vi "Convex Hull 3D (GiftWrap).vi"(0 "Vertices":sgl[][](array[numeric])=[[0.0, 0.0, 0.0], [1.0, 0.0, 0.0], [1.0, 1.0, 0.0], [0.0, 1.0, 0.0], [0.0, 0.0, 1.0], [1.0, 0.0, 1.0], [1.0, 1.0, 1.0], [0.0, 1.0, 1.0], [10.0, 10.0, 0.0], [11.0, 10.0, 0.0], [11.0, 11.0, 0.0], [10.0, 11.0, 0.0], [10.0, 10.0, 1.0], [11.0, 10.0, 1.0], [11.0, 11.0, 1.0], [10.0, 11.0, 1.0]]) -> (1 "Convex hull triangles (partial proc.)":T1[](array[typedef]), 2 "Stack error":errorcluster)   [LabVIEW 2014]
uses:
  Typedefs/Triangle.ctl
  Typedefs/Edge.ctl
  Subroutines/Cross product 3D.vi
  Subroutines/Unit vector.vi
panel:
  # "PN 21/03/2015"
  # "Vertices"
  # "Edges"
  # "Unit normal"
  # "Edge unit normals"
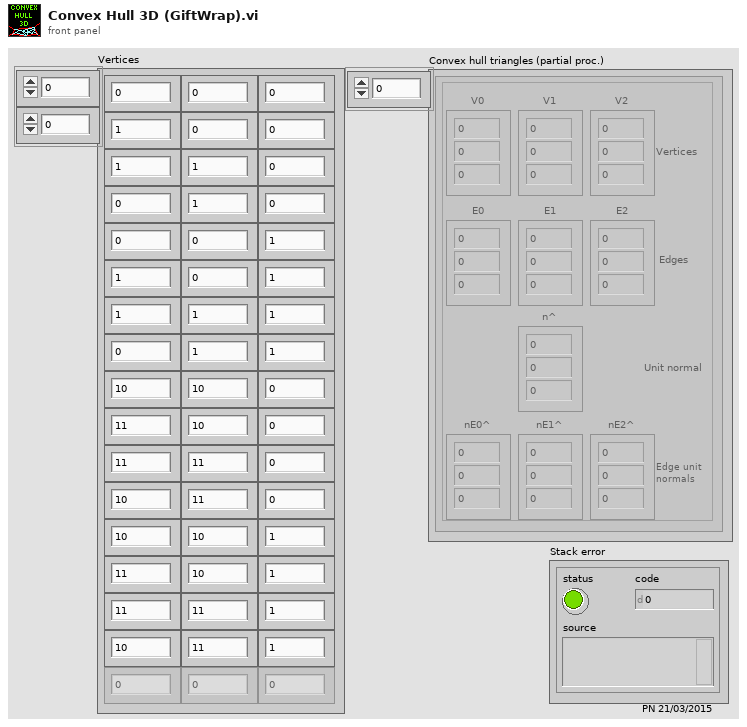
[diagram p1: front panel]
types:
  T1 = typedef "Triangle.ctl" = cluster{"V0":sgl[], "V1":sgl[], "V2":sgl[], "E0":sgl[], "E1":sgl[], "E2":sgl[], "n^":sgl[], "nE0^":sgl[], "nE1^":sgl[], "nE2^":sgl[]}
  T2 = typedef "Edge.ctl" = cluster{"V0":sgl[], "V1":sgl[], "E01":sgl[]}
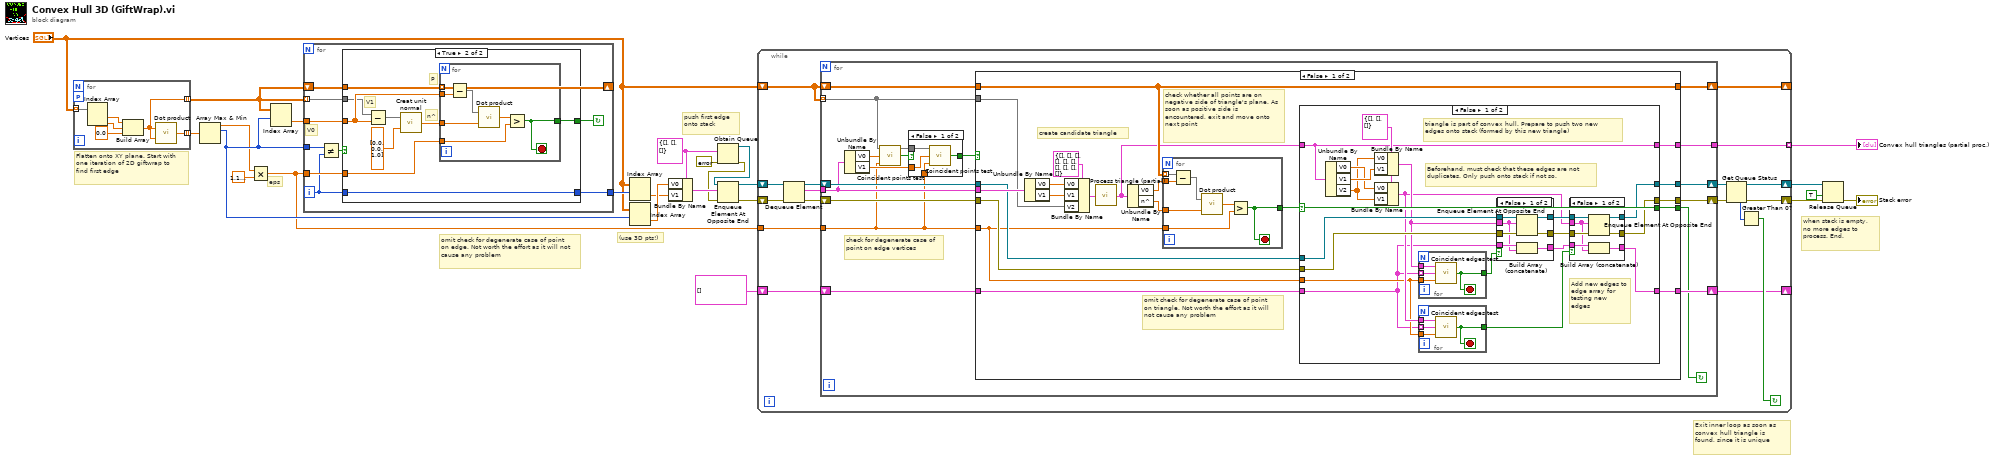
[diagram p0: block diagram]
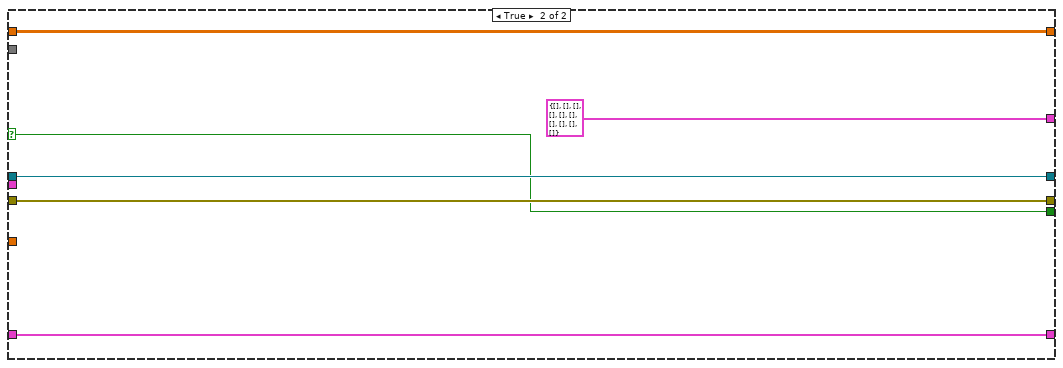
[diagram p6: hidden frame]
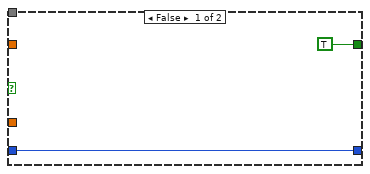
[diagram p7: hidden frame]
diagram:
  w12 = T2 {"V0"=[], "V1"=[], "E01"=[]} ("Edge")
  # "omit check for degenerate case of point on edge. Not worth the effort as it will not cause any problem"
  # "when stack is empty, no more edges to process. End."
  # "Exit inner loop as soon as convex hull triangle is found, since it is unique"
  # "(use 3D pts!)"
  # "push first edge onto stack"
  # "eps"
  # "Flatten onto XY plane. Start with one iteration of 2D giftwrap to find first edge"
  n1 = for {
    tunnel: "Vertices" -> [w30] mode=indexing
    tunnel: [w29] -> w24 mode=indexing
    workers-P: _ -> [_]
    tunnel: [w26] -> w22 mode=indexing
    n2 = Index Array(array=w30) -> (element #1=w28:sgl, element #2=w27:sgl)  [unwired: 2 in]
    n3 = Build Array(w28, w27, sgl 0.0 ("element")) -> (w26:sgl[])
    n4 = call "Dot product.vi"("B"=w26, "A"=w26) -> ("A . B"=w29:sgl)
  }
  n5 = Array Max & Min(array=w24) -> (max value=w4:sgl, max index (indices)=w13:i32)  [unwired: 2 out]
  n6 = Multiply(x=w4, y=sgl 1.1920929e-07) -> (x*y=w5:sgl)
  n7 = Index Array(array=w22, index (row)=w13) -> (element=w23:sgl[])  [unwired: 1 in]
  n8 = for {
    tunnel: w23 -> [w39]
    tunnel: w22 -> [w36] mode=indexing
    shift-right: [w37] -> _
    shift-left: w22 -> [w37]
    tunnel: w5 -> [w38]
    tunnel: [w33] -> w21
    tunnel: w13 -> [w31]
    i -> [w32]
    stop <- w35 continue-if-true
    # "V0"
    n9 = Not Equal?(x=w31, y=w32) -> (x != y?=w34:bool)
    n10 = case shown="True" w34 {
      tunnel: w39 -> [_ w48]
      tunnel: w38 -> [_ w47]
      tunnel: w37 -> [_ w46]
      tunnel: w36 -> [_ w45]
      tunnel: [TRUE w44] -> w35
      tunnel: w32 -> [w40 w42]
      tunnel: [w40 w42] -> w33
      frame False {
      }
      frame True {
        # "P"
        # "n^"
        # "V1"
        n11 = Subtract(x=w45, y=w48) -> (x-y=w43:sgl[])
        n12 = call "Creat unit normal.vi"("E2"=sgl[] [0.0, 0.0, 1.0], "E1"=w43) -> ("n^ = (E1 x E2) / ||E1 x E2||"=w49:sgl[])
        n13 = for {
          tunnel: w49 -> [w57]
          tunnel: w46 -> [w56] mode=indexing
          tunnel: w48 -> [w55]
          tunnel: w47 -> [w54]
          tunnel: [w53] -> w44
          stop <- w53 stop-if-true
          n14 = Subtract(x=w56, y=w55) -> (x-y=w52:sgl[])
          n15 = call "Dot product.vi"("B"=w57, "A"=w52) -> ("A . B"=w51:sgl)
          n16 = Greater?(x=w51, y=w54) -> (0:w53:bool)
        }
      }
    }
  }
  n17 = Index Array(array="Vertices", index (row)=w21) -> (element=w10:sgl[])  [unwired: 1 in]
  n18 = Index Array(array="Vertices", index (row)=w13) -> (element=w11:sgl[])  [unwired: 1 in]
  n19 = Bundle By Name(cluster=w12, "V0"=w11, "V1"=w10) -> (w18:T2)
  n20 = Obtain Queue(element data type=w12, error in (no error)=errorcluster {"status"=FALSE, "code"=0, "source"=""}) -> (queue out=w19:refnum<queue>, error out=w16:errorcluster)  [unwired: 3 in, 1 out]
  n21 = Enqueue Element At Opposite End(queue=w19, element=w18, error in (no error)=w16) -> (queue out=w8:refnum<queue>, error out=w9:errorcluster)  [unwired: 1 in, 1 out]
  n22 = while {
    shift-right: [w69] -> _
    shift-left: "Vertices" -> [w71]
    shift-right: [w65] -> w15
    shift-left: w8 -> [w74]
    shift-right: [w63] -> w14
    shift-left: w9 -> [w73]
    tunnel: w5 -> [w70]
    tunnel: [w60] -> w3 mode=indexing
    shift-right: [w58] -> _
    shift-left: T2[] [] -> [w59]
    stop <- w61 continue-if-true
    n23 = Dequeue Element(queue=w74, error in (no error)=w73) -> (queue out=w68:refnum<queue>, element=w72:T2, error out=w67:errorcluster)  [unwired: 1 in, 1 out]
    n24 = for {
      tunnel: w71 -> [w80] mode=indexing
      tunnel: w72 -> [w84]
      shift-right: [w90] -> w69
      shift-left: w71 -> [w91]
      tunnel: w70 -> [w78]
      shift-right: [w86] -> w66
      shift-left: w68 -> [w88]
      shift-right: [w85] -> w64
      shift-left: w67 -> [w87]
      tunnel: [w89] -> w60
      shift-right: [w76] -> w58
      shift-left: w59 -> [w77]
      stop <- w75 continue-if-true
      # "check for degenerate case of point on edge vertices"
      n25 = Unbundle By Name(w84) -> ("V0"=w83:sgl[], "V1"=w79:sgl[])
      n26 = call "Coincident points test.vi"("epsilon"=w78, "Point 2"=w83, "Point 1"=w80) -> ("Points are coincident"=w82:bool)
      n27 = case shown="False" w82 {
        selector: w82 -> [_ w96]
        tunnel: [w93 w96] -> w81
        tunnel: w80 -> [w95 _]
        tunnel: w79 -> [w94 _]
        tunnel: w78 -> [w92 _]
        frame False {
          n28 = call "Coincident points test.vi"("epsilon"=w92, "Point 2"=w94, "Point 1"=w95) -> ("Points are coincident"=w93:bool)
        }
        frame True {
        }
      }
      n29 = case shown="False" w81 {
        selector: w81 -> [_ w179]
        tunnel: w84 -> [w106 _]
        tunnel: w80 -> [w97 _]
        tunnel: w91 -> [w110 w182]
        tunnel: w78 -> [w99 _]
        tunnel: [w110 w182] -> w90
        tunnel: [w108 w179] -> w75
        tunnel: [w101 T1 {"V0"=[], "V1"=[], "V2"=[], "E0"=[], "E1"=[], "E2"=[], "n^"=[], "nE0^"=[], "nE1^"=[], "nE2^"=[]} ("Triangle out")] -> w89
        tunnel: w88 -> [w105 w181]
        tunnel: w87 -> [w107 w180]
        tunnel: [w104 w181] -> w86
        tunnel: [w103 w180] -> w85
        tunnel: w77 -> [w100 w178]
        tunnel: [w98 w178] -> w76
        frame False {
          # "omit check for degenerate case of point on triangle. Not worth the effort as it will not cause any problem"
          # "check whether all points are on negative side of triangle's plane. As soon as positive side is encountered, exit and move onto next point"
          # "create candidate triangle"
          n30 = Unbundle By Name(w106) -> ("V0"=w115:sgl[], "V1"=w114:sgl[])
          n31 = Bundle By Name(cluster=T1 {"V0"=[], "V1"=[], "V2"=[], "E0"=[], "E1"=[], "E2"=[], "n^"=[], "nE0^"=[], "nE1^"=[], "nE2^"=[]} ("Triangle"), "V0"=w115, "V1"=w114, "V2"=w97) -> (w113:T1)
          n32 = call "Process triangle (partial).vi"("Triangle in"=w113) -> ("Triangle out"=w102:T1)
          n33 = Unbundle By Name(w102) -> ("V0"=w111:sgl[], "n^"=w112:sgl[])
          n34 = for {
            tunnel: w112 -> [w176]
            tunnel: w110 -> [w175] mode=indexing
            tunnel: w111 -> [w174]
            tunnel: w99 -> [w173]
            tunnel: [w172] -> w109
            stop <- w172 stop-if-true
            n35 = Subtract(x=w175, y=w174) -> (x-y=w171:sgl[])
            n36 = call "Dot product.vi"("B"=w176, "A"=w171) -> ("A . B"=w170:sgl)
            n37 = Greater?(x=w170, y=w173) -> (0:w172:bool)
          }
          n38 = case shown="False" w109 {
            selector: w109 -> [w136 w169]
            tunnel: [w136 w169] -> w108
            tunnel: w107 -> [w131 w167]
            tunnel: w105 -> [w133 w168]
            tunnel: [w132 w168] -> w104
            tunnel: [w130 w167] -> w103
            tunnel: w102 -> [w125 w166]
            tunnel: [w125 w166] -> w101
            tunnel: w100 -> [w120 w165]
            tunnel: w99 -> [w122 _]
            tunnel: [w118 w165] -> w98
            frame False {
              w129 = T2 {"V0"=[], "V1"=[], "E01"=[]} ("Edge")
              # "Add new edges to edge array for testing new edges"
              # "Beforehand, must check that these edges are not duplicates. Only push onto stack if not so."
              # "triangle is part of convex hull. Prepare to push two new edges onto stack (formed by this new triangle)"
              n39 = Unbundle By Name(w125) -> ("V0"=w127:sgl[], "V1"=w128:sgl[], "V2"=w126:sgl[])
              n40 = Bundle By Name(cluster=w129, "V0"=w126, "V1"=w128) -> (w124:T2)
              n41 = Bundle By Name(cluster=w129, "V0"=w127, "V1"=w126) -> (w123:T2)
              n42 = for {
                tunnel: w120 -> [w164] mode=indexing
                tunnel: w124 -> [w163]
                tunnel: w122 -> [w162]
                tunnel: [w161] -> w121
                stop <- w161 stop-if-true
                n43 = call "Coincident edges test.vi"("epsilon"=w162, "Edge 2"=w164, "Edge 1"=w163) -> ("Edges are coincident"=w161:bool)
              }
              n44 = for {
                tunnel: w120 -> [w160] mode=indexing
                tunnel: w123 -> [w159]
                tunnel: w122 -> [w158]
                tunnel: [w157] -> w117
                stop <- w157 stop-if-true
                n45 = call "Coincident edges test.vi"("epsilon"=w158, "Edge 2"=w160, "Edge 1"=w159) -> ("Edges are coincident"=w157:bool)
              }
              n46 = case shown="False" w121 {
                tunnel: [w153 w156] -> w135
                tunnel: [w152 w155] -> w134
                tunnel: w133 -> [w151 w156]
                tunnel: w131 -> [w150 w155]
                tunnel: w124 -> [w148 _]
                tunnel: w120 -> [w149 w154]
                tunnel: [w147 w154] -> w119
                frame False {
                  n47 = Enqueue Element At Opposite End(queue=w151, element=w148, error in (no error)=w150) -> (queue out=w153:refnum<queue>, error out=w152:errorcluster)  [unwired: 1 in, 1 out]
                  n48 = Build Array (concatenate)(w149, w148) -> (w147:T2[])
                }
                frame True {
                }
              }
              n49 = case shown="False" w117 {
                tunnel: w135 -> [w143 w146]
                tunnel: w134 -> [w142 w145]
                tunnel: [w141 w146] -> w132
                tunnel: [w140 w145] -> w130
                tunnel: w123 -> [w138 _]
                tunnel: w119 -> [w139 w144]
                tunnel: [w137 w144] -> w118
                frame False {
                  n50 = Enqueue Element At Opposite End(queue=w143, element=w138, error in (no error)=w142) -> (queue out=w141:refnum<queue>, error out=w140:errorcluster)  [unwired: 1 in, 1 out]
                  n51 = Build Array (concatenate)(w139, w138) -> (w137:T2[])
                }
                frame True {
                }
              }
            }
            frame True {
              # "Triangle does not form the convex hull, do nothing and just move on to next point"
            }
          }
        }
        frame True {
        }
      }
    }
    n52 = Get Queue Status(queue=w66, error in (no error)=w64) -> (queue out=w65:refnum<queue>, error out=w63:errorcluster, # elements in queue=w62:i32)  [unwired: 1 in, 5 out]
    n53 = Greater Than 0?(x=w62) -> (x > 0?=w61:bool)
  }
  "Convex hull triangles (partial proc.)" <- w3
  n54 = Release Queue(queue=w15, force destroy? (F)=TRUE, error in (no error)=w14) -> (error out=→"Stack error":errorcluster)  [unwired: 2 out]
